vi "CopyFolder (subVI).vi"(3 "Boolean":bool) -> ()   [LabVIEW 2018]
panel:
  out "error out":errorcluster
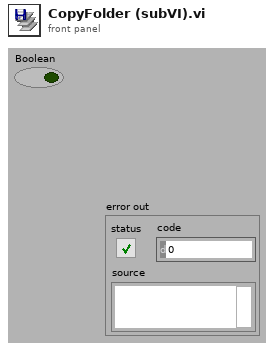
[diagram p1: front panel]
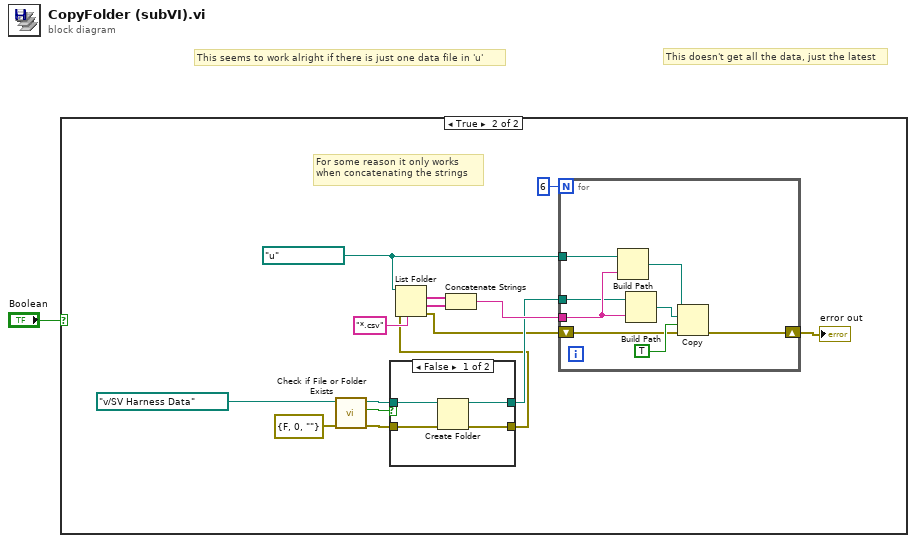
[diagram p0: block diagram]
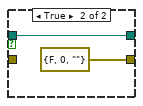
[diagram p3: hidden frame]
diagram:
  # "This doesn't get all the data, just the latest"
  # "This seems to work alright if there is just one data file in 'u'"
  n1 = case shown="True" "Boolean" {
    frame False {
    }
    frame True {
      w14 = path "u:/" ("target path (use dialog)")
      # "For some reason it only works\nwhen concatenating the strings"
      n2 = call <vilib>:"Check if File or Folder Exists.vi"("error in (no error)"=errorcluster {"status"=FALSE, "code"=0, "source"=""}, "path"=path "v:/SV Harness Data" ("target path (use dialog)")) -> ("error out"=w8:errorcluster, "file or folder exists?"=w6:bool, "dup path"=w9:path)  [unwired: 7 in]
      n3 = case shown="False" w6 {
        tunnel: [w20 w22] -> w4
        tunnel: w9 -> [w19 w22]
        tunnel: w8 -> [w18 _]
        tunnel: [w17 errorcluster {"status"=FALSE, "code"=0, "source"=""} ("error in (no error)")] -> w3
        frame False {
          n4 = Create Folder(path (use dialog)=w19, error in=w18) -> (created path=w20:path, error out=w17:errorcluster)  [unwired: 1 in, 1 out]
        }
        frame True {
        }
      }
      n5 = List Folder(path=w14, pattern="*.csv", error in=w3) -> (filenames=w12:string[], folder names=w13:string[], error out=w2:errorcluster)  [unwired: 2 out]
      n6 = Concatenate Strings(w12, w13) -> (w11:string)
      n7 = for {
        N: 6 -> [_]
        tunnel: w4 -> [w23]
        tunnel: w14 -> [w24]
        tunnel: w11 -> [w28]
        shift-right: [w29] -> w15
        shift-left: w2 -> [w25]
        n8 = Build Path(base path=w24, name or relative path=w28) -> (appended path=w26:path)
        n9 = Build Path(base path=w23, name or relative path=w28) -> (appended path=w27:path)
        n10 = Copy(8:w25, 9:TRUE ("overwrite (F)"), 10:w27, 11:w26) -> (0:w29:errorcluster)  [unwired: 1 in, 2 out]
      }
      "error out" <- w15
    }
  }
